vi "parse_duration.vi"   [LabVIEW 2012]
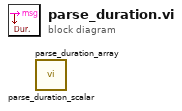
[diagram p0: block diagram]
diagram:
  n1 = call <userlib>:"parse_duration_scalar.vi"() -> ()  [unwired: 5 in, 3 out]
  n2 = call <userlib>:"parse_duration_array.vi"() -> ()  [unwired: 5 in, 3 out]
